vi "ICR_Timer_CountDown.vi"(10 "Refnum Ch":refnum<vi>, 11 "Seconds":dbl=200.0) -> ()   [LabVIEW 2015]
doc: "This VI displays the time remaining every second.\nInput parameter : the number of seconds to count down."
panel:
  out "Remaining Time":string
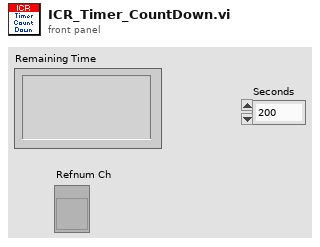
[diagram p1: front panel]
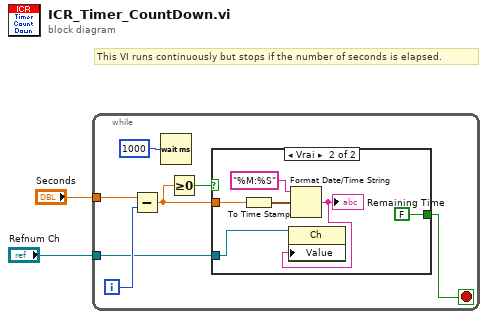
[diagram p0: block diagram]
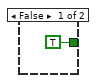
[diagram p2: hidden frame]
diagram:
  # "This VI runs continuously but stops if the number of seconds is elapsed."
  n1 = while {
    tunnel: "Seconds" -> [w7]
    tunnel: "Refnum Ch" -> [w3]
    i -> [w8]
    stop <- w4 stop-if-true
    n2 = Subtract(x=w7, y=w8) -> (x-y=w5:dbl)
    n3 = Wait (ms)(milliseconds to wait=u32 1000) -> ()  [unwired: 1 out]
    n4 = Greater Or Equal To 0?(x=w5) -> (x >= 0?=w6:bool)
    n5 = case shown="Vrai" w6 {
      tunnel: w5 -> [_ w14]
      tunnel: [TRUE FALSE] -> w4
      tunnel: w3 -> [_ w12]
      frame False {
      }
      frame True {
        n6 = To Time Stamp(1:w14) -> (0:w16:timestamp)
        n7 = Format Date/Time String(time format string (%c)="%M:%S" ("chaîne de format de l'heure (%c)"), seconds (now)=w16) -> (date/time string=w11:string)  [unwired: 1 in]
        "Remaining Time" <- w11
        n8 = property class="Ch"(reference=w12, "Value"=w11) -> ()  [unwired: 1 in, 2 out]
      }
    }
  }
